vi "DrivePath-C.vi"(11 "Params":string[][](array[string])) -> ()   [LabVIEW 2018]
uses:
  Framework/Robot Global Data.vi
  Dawgma Programming Library/Controls/PurePursuit/RobotNeededPathData.ctl
  Dawgma Programming Library/Controls/PurePursuit/PathFileData.ctl
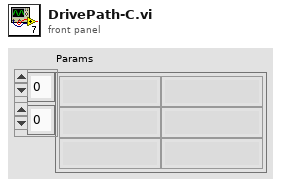
[diagram p1: front panel]
types:
  T1 = typedef "PathFileData.ctl" = cluster{"RobotNeeded":T2, "Meta":cluster{"Path (px)":cluster{i32, i32}[], "RobotWidth":dbl, "RobotLength":dbl, "CenterOfRotYOffset":dbl, "Roundedness":dbl, "StartingPositionPreset":u32}}
  T2 = typedef "RobotNeededPathData.ctl" = cluster{"Path":cluster{dbl, dbl}[], "MaxVel":dbl, "MaxAccel":dbl, "Backwards?":bool, "PointSpacing":dbl, "LookaheadDist":dbl, "Speed/Curve":dbl, "SlowDistanceAtEnd":dbl, "SlowSpeed":dbl, "MaxDeAccel":dbl}
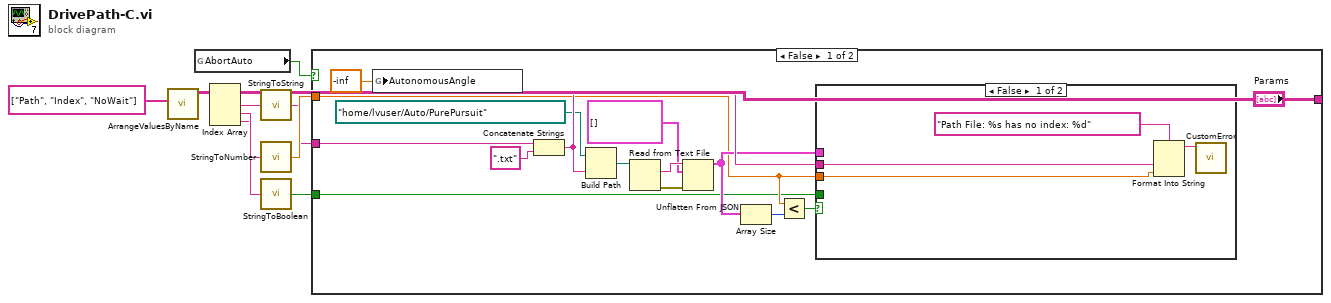
[diagram p0: block diagram]
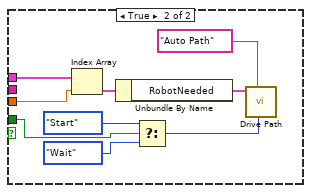
[diagram p2: hidden frame]
diagram:
  n1 = global read "Robot Global Data.vi" "AbortAuto"() -> (w10:bool)
  n2 = call "ArrangeValuesByName.vi"("Names"=string[] ["Path", "Index", "NoWait"], "Names/Values in"=w6) -> ("Values Out"=w4:string[])  [unwired: 9 in]
  n3 = Index Array(array=w4) -> (element #1=w3:string, element #2=w2:string, element #3=w1:string)  [unwired: 3 in]
  n4 = call "StringToString.vi"("String"=w3) -> ("Output"=w7:string)
  n5 = call "StringToNumber.vi"("String"=w2) -> ("Output"=w9:dbl)
  n6 = call "StringToBoolean.vi"("String"=w1) -> ("Output"=w8:bool)
  n7 = case shown="False" w10 {
    tunnel: w9 -> [w14 _]
    tunnel: w8 -> [w13 _]
    tunnel: w7 -> [w12 _]
    tunnel: ["Params" _] -> w6
    frame False {
      n8 = global write "Robot Global Data.vi" "AutonomousAngle"(-inf ("AutonomousAngle")) -> ()
      n9 = Concatenate Strings(w12, ".txt" ("string")) -> (w25:string)
      n10 = Build Path(base path=path "/home/lvuser/Auto/PurePursuit", name or relative path=w25) -> (appended path=w21:path)
      n11 = Read from Text File(file (use dialog)=w21) -> (text=w20:string, error out=w19:errorcluster)  [unwired: 3 in, 2 out]
      n12 = Unflatten From JSON(JSON string=w20, type and defaults=T1[] [], error in (no error)=w19) -> (value=w22:T1[])  [unwired: 4 in, 1 out]
      n13 = Array Size(array=w22) -> (size(s)=w23:i32)
      n14 = Less?(x=w14, y=w23) -> (x < y?=w24:bool)
      n15 = case shown="False" w24 {
        tunnel: w14 -> [w27 w38]
        tunnel: w13 -> [_ w34]
        tunnel: w22 -> [_ w30]
        tunnel: w25 -> [w26 _]
        frame False {
          n16 = Format Into String(format string="Path File: %s has no index: %d", w26, w27) -> (resulting string=w29:string)  [unwired: 2 in, 1 out]
          n17 = call "CustomError.vi"("String"=w29) -> ()  [unwired: 10 in, 1 out]
        }
        frame True {
          n18 = Index Array(array=w30, index=w38) -> (element=w37:T1)
          n19 = Unbundle By Name(w37) -> ("RobotNeeded"=w36:T2)
          n20 = Select(t=enum16{"Start", "Wait"}."Start" ("Synchronication"), s=w34, f=enum16{"Start", "Wait"}."Wait" ("Synchronication")) -> (s? t:f=w31:enum16{"Start", "Wait"})
          n21 = call "Drive Path.vi"("Synchronication"=w31, "Description"="Auto Path", "Path"=w36) -> ()  [unwired: 8 in, 1 out]
        }
      }
    }
    frame True {
    }
  }
